vi "HOST_UIC1203R.vi"() -> ()   [LabVIEW 2018]
uses:
  <instrlib>/niFgen/niFgen.llb/niFgen Output Mode.ctl
  <instrlib>/niDMM/nidmm.llb/niDMM Function.ctl
  <instrlib>/niDCPower/nidcpower.llb/niDCPower Measurement Type.ctl
  <instrlib>/niDMM/nidmm.llb/niDMM Configure Measurement Absolute.vi
panel:
  out "Power, мВт":dbl
  in  "Генератор":bool
  in  "Standard Waveform":u16(slide)=1 scale=0.0..6.0
  in  "Frequency (Hz)":dbl(knob)=50.0 min=1.0 max=100000000.0 scale=0.0..100000000.0 scale format="%_1p"
  in  "Amplitude (Vp-p)":dbl(knob)=2.4999999999999996 min=0.0 max=12.0 scale=0.0..12.0 scale format="%.1f"
  in  "DC Offset (V)":dbl(knob)=0.2 min=-6.0 max=6.0 scale=-6.0..6.0 scale format="%_1p"
  in  "FGEN Resource Name":refnum<k15>="Dev1"
  out "SEU, мВ":dbl
  in  "Instrument Descriptor":refnum<k15>="PXI1Slot5"
  in  "Питание":bool
  out "Номер образца":string="0"
  in  "SEL":path=path "C:/LabView_PRJ/23011_UIC1203R/LabView_PRJ/SEL"
  in  "DVDD_VDDA":refnum<k15>="PXI1Slot4" caption="instrument handle"
  in  "VDPIX_VCC":refnum<k15>="PXI1Slot3" caption="instrument handle"
  in  "VDA_VDD":refnum<k15>="PXI1Slot2" caption="instrument handle"
  out "VDDA Chart":dbl(graph)=0.0007214157137472484 caption="Waveform Chart 5"
  out "VDDA_cur, A":dbl caption="measurement" format="%_6g"
  in  "VDDA_curlim, A":dbl=0.1 caption="current limit" format="%_6p"
  in  "VDDA, V":dbl=1.8 caption="voltage level" format="%_6p"
  out "DVDD Chart":dbl(graph)=0.10338513624280214 caption="Waveform Chart 5"
  out "DVDD_cur, A":dbl caption="measurement" format="%_6g"
  in  "DVDD_curlim, A":dbl=0.1 caption="current limit" format="%_6p"
  in  "DVDD, V":dbl=3.3 caption="voltage level" format="%_6p"
  out "VCC Chart":dbl(graph)=-0.0011085533359822216
  out "VCC_cur, A":dbl caption="measurement" format="%_6g"
  in  "VCC, V":dbl=3.3 caption="voltage level" format="%_6p"
  in  "VCC_curlim, A":dbl=0.1 caption="current limit" format="%_6p"
  out "VDA Chart":dbl(graph)=-0.15026988538913832 caption="Waveform Chart 5"
  out "VDPIX Chart":dbl(graph)=0.2888581876247902
  out "VDD Chart":dbl(graph)=-0.0007912650485297681
  out "VDPIX_cur, A":dbl caption="measurement" format="%_6g"
  in  "VDPIX_curlim, A":dbl=0.1 caption="current limit" format="%_6p"
  in  "VDPIX, V":dbl=1.8 caption="voltage level" format="%_6p"
  in  "VDD, V":dbl=1.8 caption="voltage level" format="%_6p"
  out "VDD_cur, A":dbl caption="measurement" format="%_6g"
  out "VDA_cur, A":dbl caption="measurement" format="%_6g"
  in  "VDD_curlim, A":dbl=0.1 caption="current limit" format="%_6p"
  in  "VDA_curlim, A":dbl=0.1 caption="current limit" format="%_6p"
  in  "VDA, V":dbl=1.8 caption="voltage level" format="%_6p"
  in  "Стоп":bool
  in  "Период, мс":u32=100
  out "DVDD":bool
  out "DVDD":i32
  in  "DVDD_selcur":dbl=0.095 caption="current limit" format="%_6p"
  out "VCC":bool
  out "VCC":i32
  in  "VCC_selcur":dbl=0.095 caption="current limit" format="%_6p"
  out "VDPIX":bool
  out "VDPIX":i32
  out "VDD":bool
  out "VDD":i32
  out "VDA":bool
  out "VDA":i32
  in  "VDPIX_selcur":dbl=0.095 caption="current limit" format="%_6p"
  in  "VDD_selcur":dbl=0.095 caption="current limit" format="%_6p"
  in  "VDA_selcur":dbl=0.095 caption="current limit" format="%_6p"
  out "SEL":bool
  in  "SIM_SEL":bool
  out "VDDA":bool
  out "VDDA":i32
  in  "VDDA_selcur":dbl=0.095 caption="current limit" format="%_6p"
  # "2"
  # "1"
  # "3"
  # "Гц"
  # "Амплитуда"
  # "Смещение"
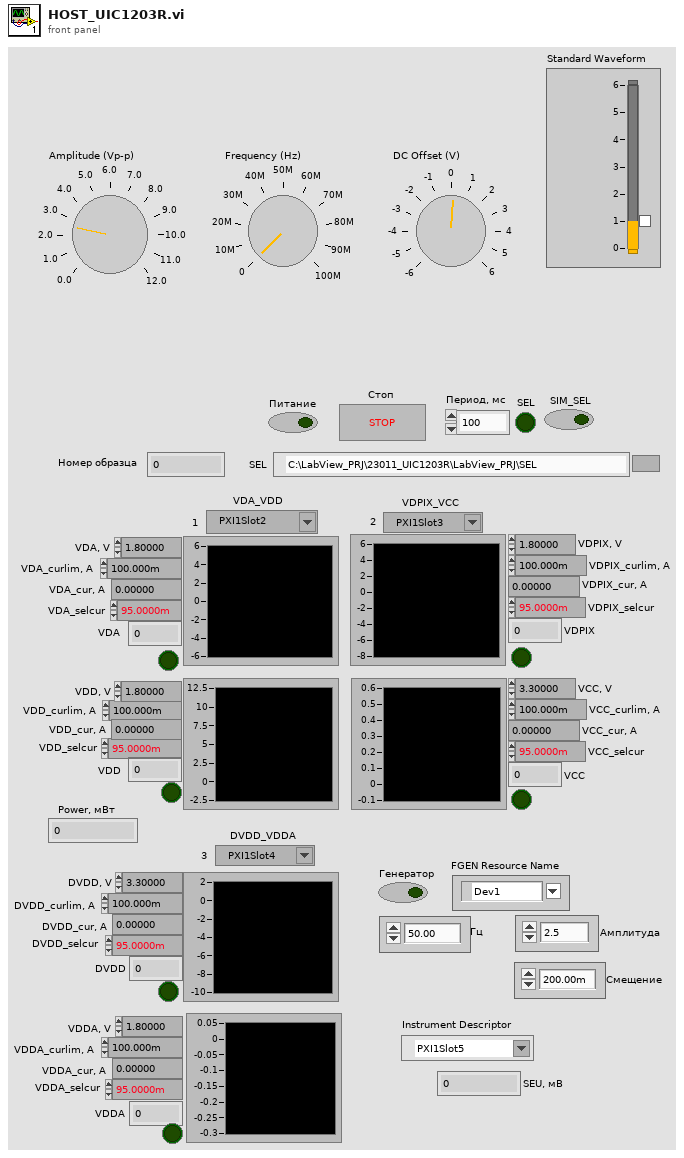
[diagram p1: front panel]
types:
  T1 = typedef "niFgen Output Mode.ctl" = u32
  T2 = enum16{"open", "replace", "create", "open or create", "replace or create", "replace or create with confirmation"}
  T3 = typedef "niDCPower Measurement Type.ctl" = i32
  T4 = typedef "niDMM Function.ctl" = enum16{"DC Volts", "AC Volts", "DC Current", "AC Current", "2-wire Resistance", "4-wire Resistance", "Diode", "Frequency", "Period", "AC Volts DC Coupled", "Capacitance", "Inductance", "Temperature"}
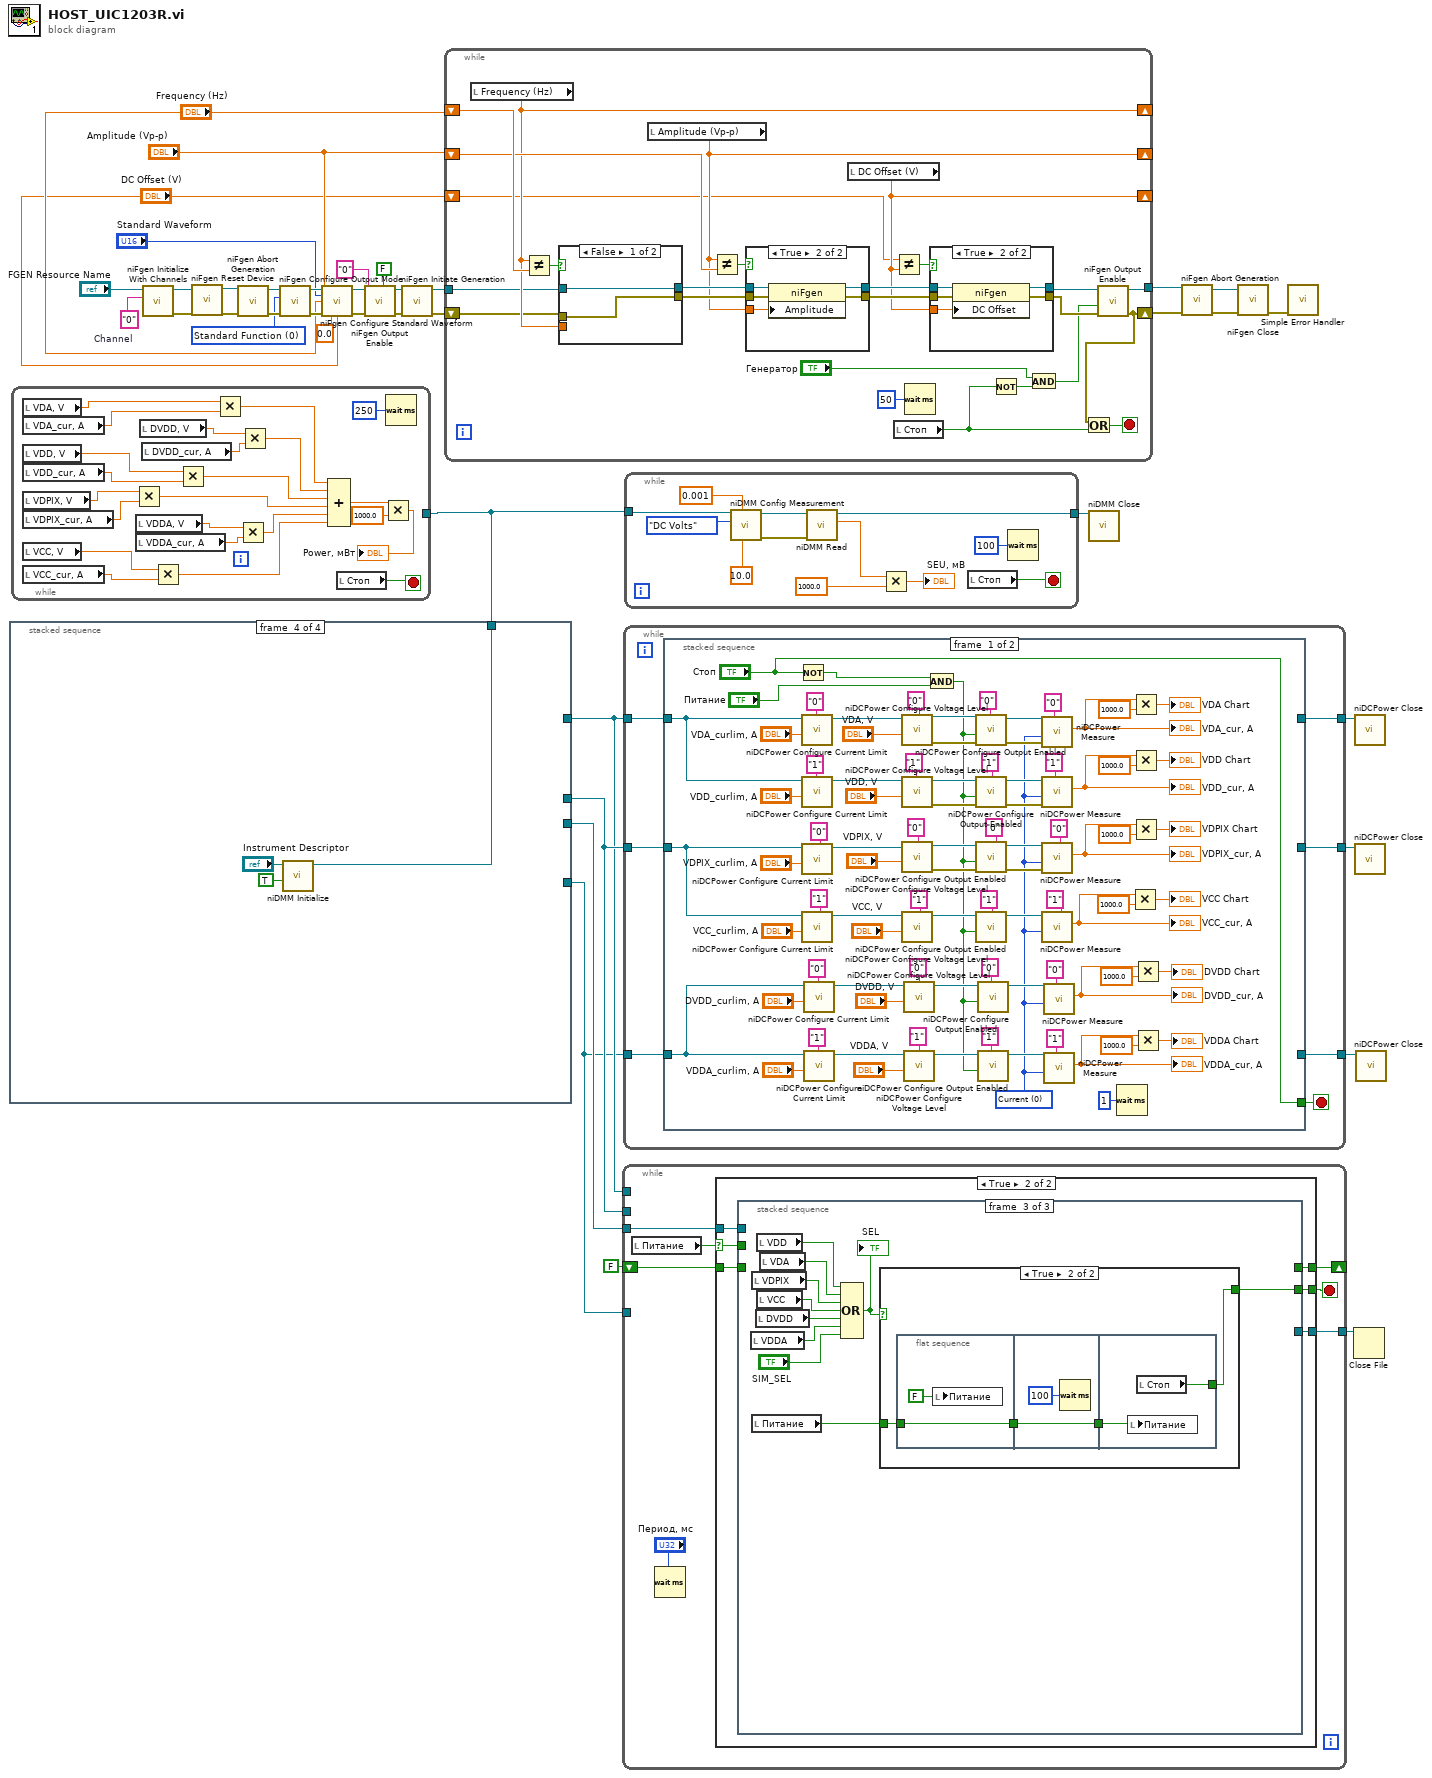
[diagram p0: block diagram]
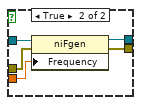
[diagram p4: hidden frame]
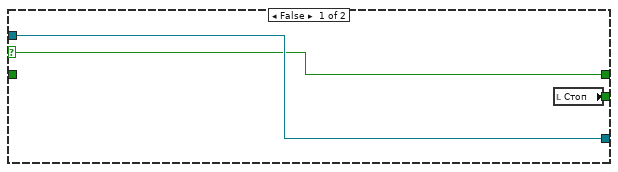
[diagram p5: hidden frame]
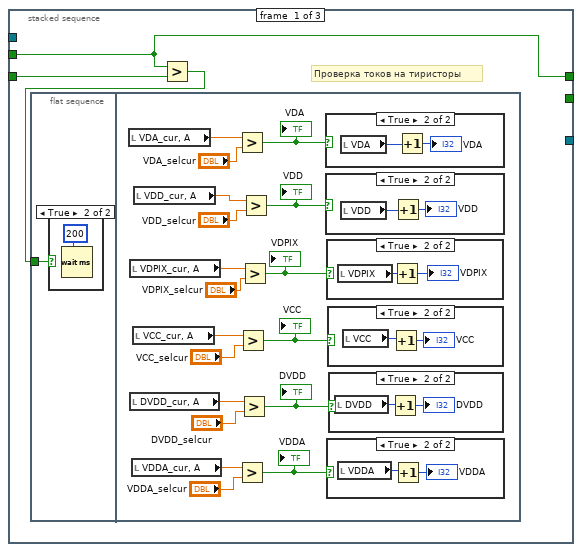
[diagram p6: hidden frame]
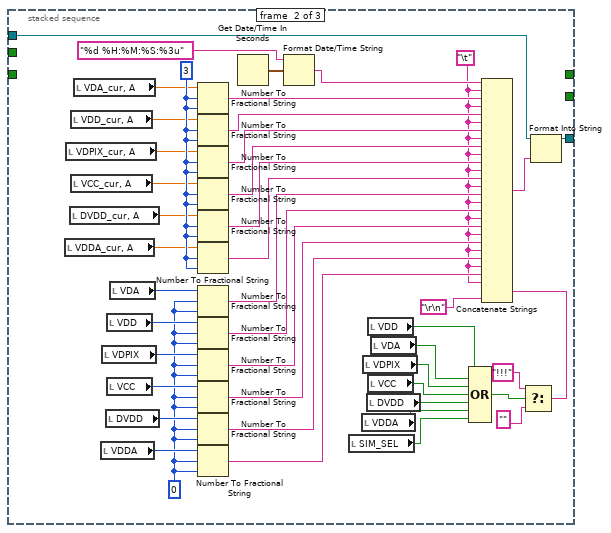
[diagram p14: hidden frame]
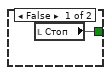
[diagram p15: hidden frame]
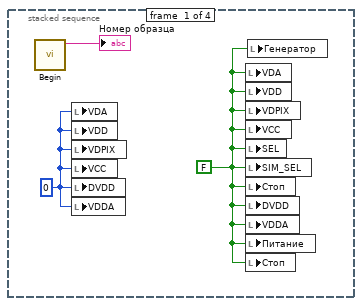
[diagram p17: hidden frame]
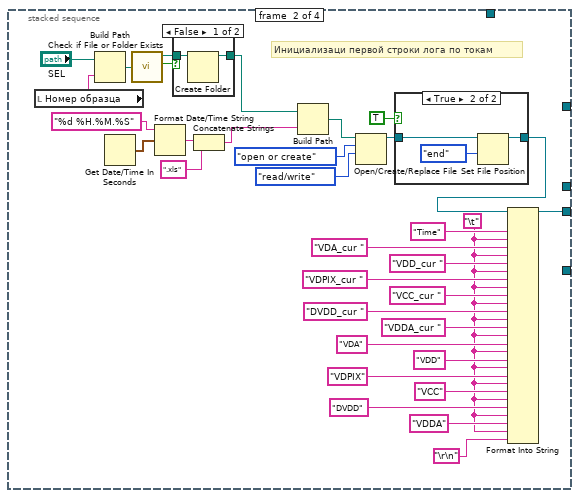
[diagram p18: hidden frame]
diagram:
  w20 = T1 0 items=["Standard Function", "Frequency List", "Arbitrary Waveform", "Arbitrary Sequence", "Script"] ("output mode")
  w9 = "0"  # Channel
  n1 = stacked-sequence {
    tunnel: [_ _ w94 _] -> w37
    tunnel: [_ _ w93 _] -> w36
    tunnel: [_ w60 _ _] -> w39
    tunnel: [_ _ w87 _] -> w32
    tunnel: [_ _ _ w105] -> w1
    frame #0 {
      w42 = 0
      w41 = FALSE
      n2 = call "Begin.vi"() -> ("Номер образца 2"=→"Номер образца":string)  [unwired: 11 in]
      n3 = local write "VDA"(w42) -> ()
      n4 = local write "VDD"(w42) -> ()
      n5 = local write "VDPIX"(w42) -> ()
      n6 = local write "VCC"(w42) -> ()
      n7 = local write "DVDD"(w42) -> ()
      n8 = local write "VDDA"(w42) -> ()
      n9 = local write "VDA"(w41) -> ()
      n10 = local write "VDD"(w41) -> ()
      n11 = local write "VDPIX"(w41) -> ()
      n12 = local write "VCC"(w41) -> ()
      n13 = local write "SEL"(w41) -> ()
      n14 = local write "SIM_SEL"(w41) -> ()
      n15 = local write "Стоп"(w41) -> ()
      n16 = local write "DVDD"(w41) -> ()
      n17 = local write "VDDA"(w41) -> ()
      n18 = local write "Питание"(w41) -> ()
      n19 = local write "Стоп"(w41) -> ()
      n20 = local write "Генератор"(w41) -> ()
    }
    frame #1 {
      w45 = "\t"
      # "Инициализаци первой строки лога по токам"
      n21 = local read "Номер образца"() -> (w72:string)
      n22 = Build Path(base path="SEL", name or relative path=w72) -> (appended path=w74:path)
      n23 = Get Date/Time In Seconds() -> (seconds since 1Jan1904=w67:timestamp)
      n24 = call <vilib>:"Check if File or Folder Exists.vi"("path"=w74) -> ("file or folder exists?"=w75:bool, "dup path"=w76:path)  [unwired: 8 in, 1 out]
      n25 = Format Date/Time String(time format string (%c)="%d %H.%M.%S", seconds (now)=w67) -> (date/time string=w64:string)  [unwired: 1 in]
      n26 = case shown="False" w75 {
        tunnel: w76 -> [w82 w83]
        tunnel: [w81 w83] -> w59
        frame False {
          n27 = Create Folder(path (use dialog)=w82) -> (created path=w81:path)  [unwired: 2 in, 2 out]
        }
        frame True {
        }
      }
      n28 = Concatenate Strings(w64, ".xls" ("string")) -> (w62:string)
      n29 = Build Path(base path=w59, name or relative path=w62) -> (appended path=w65:path)
      n30 = Open/Create/Replace File(file path (use dialog)=w65, operation (0:open)=T2."open or create", access (0:read/write)=enum16{"read/write", "read-only", "write-only"}."read/write") -> (refnum out=w68:refnum<file>)  [unwired: 3 in, 2 out]
      n31 = case shown="True" TRUE {
        tunnel: w68 -> [w77 w80]
        tunnel: [w77 w78] -> w61
        frame False {
        }
        frame True {
          n32 = Set File Position(refnum=w80, from (0:start)=enum16{"start", "end", "current"}."end") -> (refnum out=w78:refnum<file>)  [unwired: 2 in, 1 out]
        }
      }
      n33 = Format Into String(initial string=w61, "Time" ("input 1"), w45, "VDA_cur " ("input 1"), w45, "VDD_cur " ("input 1"), w45, "VDPIX_cur " ("input 1"), w45, "VCC_cur " ("input 1"), w45, "DVDD_cur " ("input 1"), w45, "VDDA_cur " ("input 1"), w45, "VDA" ("input 1"), w45, "VDD" ("input 1"), w45, "VDPIX" ("input 1"), w45, "VCC" ("input 1"), w45, "DVDD" ("input 1"), w45, "VDDA" ("input 1"), w45, "\r\n") -> (resulting string=w60:refnum<file>)  [unwired: 2 in, 1 out]
    }
    frame #2 {
      n34 = call <instrlib>:"niDCPower Initialize.vi"("reset device"=TRUE, "resource name"="DVDD_VDDA") -> ("error out"=w90:errorcluster, "instrument handle out"=w89:refnum<k15>)  [unwired: 2 in, 6 out]
      n35 = call <instrlib>:"niDCPower Initialize.vi"("reset device"=TRUE, "resource name"="VDA_VDD") -> ("error out"=w101:errorcluster, "instrument handle out"=w103:refnum<k15>)  [unwired: 2 in, 6 out]
      n36 = call <instrlib>:"niDCPower Initialize.vi"("reset device"=TRUE, "resource name"="VDPIX_VCC") -> ("error out"=w102:errorcluster, "instrument handle out"=w104:refnum<k15>)  [unwired: 2 in, 6 out]
      n37 = call <instrlib>:"niDCPower Configure Voltage Level.vi"("error in (no error)"=w101, "voltage level"=0.0, "channel name"="0,1", "instrument handle"=w103) -> ("instrument handle out"=w93:refnum<k15>)  [unwired: 6 in, 1 out]
      n38 = call <instrlib>:"niDCPower Configure Voltage Level.vi"("error in (no error)"=w102, "voltage level"=0.0, "channel name"="0,1", "instrument handle"=w104) -> ("instrument handle out"=w94:refnum<k15>)  [unwired: 6 in, 1 out]
      n39 = call <instrlib>:"niDCPower Configure Voltage Level.vi"("error in (no error)"=w90, "voltage level"=0.0, "channel name"="0,1", "instrument handle"=w89) -> ("instrument handle out"=w87:refnum<k15>)  [unwired: 6 in, 1 out]
    }
    frame #3 {
      n40 = call <instrlib>:"niDMM Initialize.vi"("Reset"=TRUE, "Instrument Descriptor"="Instrument Descriptor") -> ("instrument handle out"=w105:refnum<k15>)  [unwired: 8 in, 1 out]
    }
  }
  n41 = while {
    tunnel: w1 -> [_]
    stop <- w130 stop-if-true
    n42 = local read "VDA, V"() -> (w126:dbl)
    n43 = local read "VDA_cur, A"() -> (w125:dbl)
    n44 = local read "VDD, V"() -> (w122:dbl)
    n45 = local read "VDD_cur, A"() -> (w121:dbl)
    n46 = local read "VDPIX, V"() -> (w127:dbl)
    n47 = local read "VDPIX_cur, A"() -> (w128:dbl)
    n48 = local read "VCC, V"() -> (w120:dbl)
    n49 = local read "VCC_cur, A"() -> (w119:dbl)
    n50 = Multiply(x=w127, y=w128) -> (x*y=w113:dbl)
    n51 = local read "VDDA, V"() -> (w118:dbl)
    n52 = local read "VDDA_cur, A"() -> (w117:dbl)
    n53 = local read "DVDD, V"() -> (w124:dbl)
    n54 = local read "DVDD_cur, A"() -> (w123:dbl)
    n55 = Multiply(x=w120, y=w119) -> (x*y=w111:dbl)
    n56 = Multiply(x=w122, y=w121) -> (x*y=w114:dbl)
    n57 = Multiply(x=w126, y=w125) -> (x*y=w116:dbl)
    n58 = Multiply(x=w118, y=w117) -> (x*y=w112:dbl)
    n59 = Multiply(x=w124, y=w123) -> (x*y=w115:dbl)
    n60 = Compound Arithmetic op=ADD(w116, w115, w114, w113, w112, w111) -> (w110:dbl)
    n61 = local read "Стоп"() -> (w130:bool)
    n62 = Multiply(x=w110, y=1000.0) -> (x*y=→"Power, мВт":dbl)
    n63 = Wait (ms)(milliseconds to wait=u32 250) -> ()  [unwired: 1 out]
  }
  n64 = call <instrlib>:"niFgen Initialize With Channels.vi"("Channel Name"=w9, "Resource Name"="FGEN Resource Name") -> ("error out"=w2:errorcluster, "Instrument Handle Out"=w5:refnum<k15>)  [unwired: 8 in]
  n65 = call <instrlib>:"niFgen Reset Device.vi"("error in (no error)"=w2, "Instrument Handle"=w5) -> ("error out"=w3:errorcluster, "Instrument Handle Out"=w4:refnum<k15>)  [unwired: 8 in]
  n66 = call <instrlib>:"niFgen Abort Generation.vi"("error in (no error)"=w3, "Instrument Handle"=w4) -> ("error out"=w23:errorcluster, "Instrument Handle Out"=w22:refnum<k15>)  [unwired: 8 in]
  n67 = call <instrlib>:"niFgen Configure Output Mode.vi"("error in (no error)"=w23, "Output Mode (default: 0=Standard Function)"=w20, "Instrument Handle"=w22) -> ("error out"=w27:errorcluster, "Instrument Handle Out"=w25:refnum<k15>)  [unwired: 6 in]
  n68 = call <instrlib>:"niFgen Configure Standard Waveform.vi"("Instrument Handle"=w25, "Waveform"="Standard Waveform", "Frequency"="Frequency (Hz)", "Amplitude"="Amplitude (Vp-p)", "error in (no error)"=w27, "Start Phase"=0.0, "DC Offset"="DC Offset (V)") -> ("Instrument Handle Out"=w18:refnum<k15>, "error out"=w19:errorcluster)  [unwired: 7 in]
  n69 = call <instrlib>:"niFgen Output Enable.vi"("error in (no error)"=w19, "Output Enable (default: True)"=FALSE ("output enable"), "Channel Name"="0", "Instrument Handle"=w18) -> ("error out"=w26:errorcluster, "Instrument Handle Out"=w24:refnum<k15>)  [unwired: 6 in]
  n70 = call <instrlib>:"niFgen Initiate Generation.vi"("error in (no error)"=w26, "Instrument Handle"=w24) -> ("error out"=w13:errorcluster, "Instrument Handle Out"=w17:refnum<k15>)  [unwired: 8 in]
  n71 = while {
    tunnel: w17 -> [w131]
    tunnel: [w140] -> w16
    shift-right: [w144] -> _
    shift-left: "Frequency (Hz)" -> [w151]
    shift-right: [w143] -> _
    shift-left: "Amplitude (Vp-p)" -> [w150]
    shift-right: [w142] -> _
    shift-left: "DC Offset (V)" -> [w141]
    shift-right: [w136] -> w12
    shift-left: w13 -> [w132]
    stop <- w145 stop-if-true
    n72 = local read "Frequency (Hz)"() -> (w144:dbl)
    n73 = Not Equal?(x=w144, y=w151) -> (x != y?=w149:bool)
    n74 = case shown="False" w149 {
      tunnel: [w171 w176] -> w152
      tunnel: [w170 w175] -> w153
      tunnel: w131 -> [w171 w174]
      tunnel: w144 -> [_ w173]
      tunnel: w132 -> [w170 w172]
      frame False {
      }
      frame True {
        n75 = property class="niFgen"(reference=w174, error in=w172, "Frequency"=w173) -> (reference out=w176:refnum<k15>, error out=w175:errorcluster)
      }
    }
    n76 = local read "Amplitude (Vp-p)"() -> (w143:dbl)
    n77 = Not Equal?(x=w143, y=w150) -> (x != y?=w148:bool)
    n78 = case shown="True" w148 {
      tunnel: w152 -> [w164 w169]
      tunnel: w153 -> [w163 w168]
      tunnel: [w163 w167] -> w154
      tunnel: [w164 w166] -> w155
      tunnel: w143 -> [_ w165]
      frame False {
      }
      frame True {
        n79 = property class="niFgen"(reference=w169, error in=w168, "Amplitude"=w165) -> (reference out=w166:refnum<k15>, error out=w167:errorcluster)
      }
    }
    n80 = local read "DC Offset (V)"() -> (w142:dbl)
    n81 = Not Equal?(x=w141, y=w142) -> (x != y?=w147:bool)
    n82 = local read "Стоп"() -> (w134:bool)
    n83 = Wait (ms)(milliseconds to wait=u32 50) -> ()  [unwired: 1 out]
    n84 = case shown="True" w147 {
      tunnel: w154 -> [w156 w162]
      tunnel: w155 -> [w157 w161]
      tunnel: [w157 w160] -> w139
      tunnel: [w156 w159] -> w138
      tunnel: w142 -> [_ w158]
      frame False {
      }
      frame True {
        n85 = property class="niFgen"(reference=w161, error in=w162, "DC Offset"=w158) -> (reference out=w160:refnum<k15>, error out=w159:errorcluster)
      }
    }
    n86 = Not(x=w134) -> (.not. x?=w137:bool)
    n87 = And(x="Генератор", y=w137) -> (x .and. y?=w133:bool)
    n88 = call <instrlib>:"niFgen Output Enable.vi"("error in (no error)"=w138, "Output Enable (default: True)"=w133, "Instrument Handle"=w139) -> ("error out"=w136:errorcluster, "Instrument Handle Out"=w140:refnum<k15>)  [unwired: 7 in]
    n89 = Or(x=w136, y=w134) -> (x .or. y?=w145:bool)
  }
  n90 = while {
    shift-right: [w177] -> _
    shift-left: FALSE -> [w183]
    tunnel: w39 -> [w182]
    tunnel: [w180] -> w38
    tunnel: w32 -> [_]
    tunnel: w37 -> [_]
    tunnel: w36 -> [_]
    stop <- w181 stop-if-true
    n91 = local read "Питание"() -> (w178:bool)
    n92 = Wait (ms)(milliseconds to wait="Период, мс") -> ()  [unwired: 1 out]
    n93 = case shown="True" w178 {
      selector: w178 -> [w184 w188]
      tunnel: w183 -> [_ w192]
      tunnel: w182 -> [w185 w191]
      tunnel: [w186 w190] -> w181
      tunnel: [w185 w189] -> w180
      tunnel: [w184 w187] -> w177
      frame False {
        n94 = local read "Стоп"() -> (w186:bool)
      }
      frame True {
        n95 = stacked-sequence {
          tunnel: w192 -> [w195 _ _]
          tunnel: w191 -> [_ w262 _]
          tunnel: [_ _ w274] -> w190
          tunnel: [_ w260 _] -> w189
          tunnel: w188 -> [w194 _ _]
          tunnel: [w194 _ _] -> w187
          frame #0 {
            # "Проверка токов на тиристоры"
            n96 = flat-sequence {
              tunnel: w193 -> [w196]
              frame #0 {
                n97 = case shown="True" w196 {
                  frame False {
                  }
                  frame True {
                    n98 = Wait (ms)(milliseconds to wait=u32 200) -> ()  [unwired: 1 out]
                  }
                }
              }
              frame #1 {
                n99 = local read "VDA_cur, A"() -> (w209:dbl)
                n100 = local read "VDPIX_cur, A"() -> (w207:dbl)
                n101 = local read "DVDD_cur, A"() -> (w201:dbl)
                n102 = local read "VDDA_cur, A"() -> (w198:dbl)
                n103 = local read "VCC_cur, A"() -> (w206:dbl)
                n104 = local read "VDD_cur, A"() -> (w208:dbl)
                n105 = Greater?(x=w209, y="VDA_selcur") -> (0:w214:bool)
                "VDA" <- w214
                n106 = Greater?(x=w198, y="VDDA_selcur") -> (0:w200:bool)
                "VDDA" <- w200
                n107 = Greater?(x=w206, y="VCC_selcur") -> (0:w205:bool)
                "VCC" <- w205
                n108 = Greater?(x=w201, y="DVDD_selcur") -> (0:w202:bool)
                "DVDD" <- w202
                n109 = Greater?(x=w207, y="VDPIX_selcur") -> (0:w210:bool)
                "VDPIX" <- w210
                n110 = Greater?(x=w208, y="VDD_selcur") -> (0:w212:bool)
                "VDD" <- w212
                n111 = case shown="True" w214 {
                  frame False {
                  }
                  frame True {
                    n112 = local read "VDA"() -> (w227:i32)
                    n113 = Increment(x=w227) -> (x+1=→"VDA":i32)
                  }
                }
                n114 = case shown="True" w212 {
                  frame False {
                  }
                  frame True {
                    n115 = local read "VDD"() -> (w224:i32)
                    n116 = Increment(x=w224) -> (x+1=→"VDD":i32)
                  }
                }
                n117 = case shown="True" w210 {
                  frame False {
                  }
                  frame True {
                    n118 = local read "VDPIX"() -> (w223:i32)
                    n119 = Increment(x=w223) -> (x+1=→"VDPIX":i32)
                  }
                }
                n120 = case shown="True" w200 {
                  frame False {
                  }
                  frame True {
                    n121 = local read "VDDA"() -> (w217:i32)
                    n122 = Increment(x=w217) -> (x+1=→"VDDA":i32)
                  }
                }
                n123 = case shown="True" w205 {
                  frame False {
                  }
                  frame True {
                    n124 = local read "VCC"() -> (w221:i32)
                    n125 = Increment(x=w221) -> (x+1=→"VCC":i32)
                  }
                }
                n126 = case shown="True" w202 {
                  frame False {
                  }
                  frame True {
                    n127 = local read "DVDD"() -> (w219:i32)
                    n128 = Increment(x=w219) -> (x+1=→"DVDD":i32)
                  }
                }
              }
            }
            n129 = Greater?(x=w194, y=w195) -> (0:w193:bool)
          }
          frame #1 {
            w230 = i16 0 ("width (-)")
            w259 = i16 3 ("width (-)")
            w231 = "\t"
            n130 = local read "VDDA_cur, A"() -> (w250:dbl)
            n131 = local read "VDPIX_cur, A"() -> (w253:dbl)
            n132 = local read "DVDD_cur, A"() -> (w251:dbl)
            n133 = local read "VDD_cur, A"() -> (w254:dbl)
            n134 = local read "VCC_cur, A"() -> (w252:dbl)
            n135 = local read "VDA_cur, A"() -> (w255:dbl)
            n136 = local read "VDDA"() -> (w240:i32)
            n137 = local read "VDPIX"() -> (w247:i32)
            n138 = local read "DVDD"() -> (w245:i32)
            n139 = local read "VDD"() -> (w248:i32)
            n140 = local read "VCC"() -> (w246:i32)
            n141 = local read "VDA"() -> (w249:i32)
            n142 = Number To Fractional String(number=w255, width (-)=w259, precision (6)=w259) -> (F-format string=w266:string)  [unwired: 1 in]
            n143 = Number To Fractional String(number=w254, width (-)=w259, precision (6)=w259) -> (F-format string=w265:string)  [unwired: 1 in]
            n144 = Number To Fractional String(number=w253, width (-)=w259, precision (6)=w259) -> (F-format string=w264:string)  [unwired: 1 in]
            n145 = Number To Fractional String(number=w252, width (-)=w259, precision (6)=w259) -> (F-format string=w261:string)  [unwired: 1 in]
            n146 = Number To Fractional String(number=w251, width (-)=w259, precision (6)=w259) -> (F-format string=w257:string)  [unwired: 1 in]
            n147 = Number To Fractional String(number=w250, width (-)=w259, precision (6)=w259) -> (F-format string=w256:string)  [unwired: 1 in]
            n148 = Number To Fractional String(number=w249, width (-)=w230, precision (6)=w230) -> (F-format string=w237:string)  [unwired: 1 in]
            n149 = Number To Fractional String(number=w248, width (-)=w230, precision (6)=w230) -> (F-format string=w236:string)  [unwired: 1 in]
            n150 = Number To Fractional String(number=w247, width (-)=w230, precision (6)=w230) -> (F-format string=w235:string)  [unwired: 1 in]
            n151 = Number To Fractional String(number=w246, width (-)=w230, precision (6)=w230) -> (F-format string=w234:string)  [unwired: 1 in]
            n152 = Number To Fractional String(number=w245, width (-)=w230, precision (6)=w230) -> (F-format string=w233:string)  [unwired: 1 in]
            n153 = Number To Fractional String(number=w240, width (-)=w230, precision (6)=w230) -> (F-format string=w232:string)  [unwired: 1 in]
            n154 = Get Date/Time In Seconds() -> (seconds since 1Jan1904=w272:timestamp)
            n155 = Format Date/Time String(time format string (%c)="%d %H:%M:%S:%3u", seconds (now)=w272) -> (date/time string=w267:string)  [unwired: 1 in]
            n156 = local read "SIM_SEL"() -> (w238:bool)
            n157 = local read "VDDA"() -> (w239:bool)
            n158 = local read "VDPIX"() -> (w242:bool)
            n159 = local read "DVDD"() -> (w258:bool)
            n160 = local read "VDD"() -> (w244:bool)
            n161 = local read "VCC"() -> (w241:bool)
            n162 = local read "VDA"() -> (w243:bool)
            n163 = Compound Arithmetic op=OR(w244, w243, w242, w241, w258, w239, w238) -> (w263:bool)
            n164 = Select(t="!!!", s=w263, f="") -> (s? t:f=w229:string)
            n165 = Concatenate Strings(w267, w231, w266, w231, w265, w231, w264, w231, w261, w231, w257, w231, w256, w231, w237, w231, w236, w231, w235, w231, w234, w231, w233, w231, w232, w231, w229, "\r\n") -> (w271:string)
            n166 = Format Into String(initial string=w262, w271) -> (resulting string=w260:refnum<file>)  [unwired: 2 in, 1 out]
          }
          frame #2 {
            n167 = local read "VDDA"() -> (w276:bool)
            n168 = local read "VDPIX"() -> (w278:bool)
            n169 = local read "Питание"() -> (w273:bool)
            n170 = local read "DVDD"() -> (w282:bool)
            n171 = local read "VDD"() -> (w280:bool)
            n172 = local read "VCC"() -> (w277:bool)
            n173 = local read "VDA"() -> (w279:bool)
            n174 = Compound Arithmetic op=OR(w280, w279, w278, w277, w282, w276, "SIM_SEL") -> (w281:bool)
            "SEL" <- w281
            n175 = case shown="True" w281 {
              tunnel: [w283 w284] -> w274
              tunnel: w273 -> [_ w285]
              frame False {
                n176 = local read "Стоп"() -> (w283:bool)
              }
              frame True {
                n177 = flat-sequence {
                  tunnel: [w288] -> w286
                  tunnel: w285 -> [w288]
                  tunnel: [w290] -> w287
                  tunnel: w286 -> [w290]
                  tunnel: w287 -> [w293]
                  tunnel: [w292] -> w284
                  frame #0 {
                    n178 = local write "Питание"(FALSE ("Питание")) -> ()
                  }
                  frame #1 {
                    n179 = Wait (ms)(milliseconds to wait=u32 100) -> ()  [unwired: 1 out]
                  }
                  frame #2 {
                    n180 = local write "Питание"(w293) -> ()
                    n181 = local read "Стоп"() -> (w292:bool)
                  }
                }
              }
            }
          }
        }
      }
    }
  }
  n182 = while {
    tunnel: w36 -> [w300]
    tunnel: w32 -> [w298]
    tunnel: w37 -> [w299]
    tunnel: [w297] -> w35
    tunnel: [w296] -> w34
    tunnel: [w295] -> w33
    stop <- w294 stop-if-true
    n183 = stacked-sequence {
      tunnel: w298 -> [w307 w388]
      tunnel: w299 -> [w306 w389]
      tunnel: w300 -> [w305 w390]
      tunnel: [_ w390] -> w297
      tunnel: [_ w389] -> w296
      tunnel: [_ w388] -> w295
      tunnel: ["Стоп" _] -> w294
      frame #0 {
        w308 = T3 0 items=["Current", "Voltage"] ("measurement type")
        n184 = Not(x="Стоп") -> (.not. x?=w302:bool)
        n185 = call <instrlib>:"niDCPower Configure Current Limit.vi"("current limit"="VDA_curlim, A", "channel name"="0", "instrument handle"=w305) -> ("instrument handle out"=w376:refnum<k15>)  [unwired: 7 in, 1 out]
        n186 = call <instrlib>:"niDCPower Configure Current Limit.vi"("current limit"="VDD_curlim, A", "channel name"="1", "instrument handle"=w305) -> ("instrument handle out"=w377:refnum<k15>)  [unwired: 7 in, 1 out]
        n187 = call <instrlib>:"niDCPower Configure Current Limit.vi"("current limit"="VDPIX_curlim, A", "channel name"="0", "instrument handle"=w306) -> ("instrument handle out"=w359:refnum<k15>)  [unwired: 7 in, 1 out]
        n188 = call <instrlib>:"niDCPower Configure Current Limit.vi"("current limit"="VCC_curlim, A", "channel name"="1", "instrument handle"=w306) -> ("instrument handle out"=w339:refnum<k15>)  [unwired: 7 in, 1 out]
        n189 = call <instrlib>:"niDCPower Configure Current Limit.vi"("current limit"="DVDD_curlim, A", "channel name"="0", "instrument handle"=w307) -> ("instrument handle out"=w330:refnum<k15>)  [unwired: 7 in, 1 out]
        n190 = call <instrlib>:"niDCPower Configure Current Limit.vi"("current limit"="VDDA_curlim, A", "channel name"="1", "instrument handle"=w307) -> ("instrument handle out"=w311:refnum<k15>)  [unwired: 7 in, 1 out]
        n191 = call <instrlib>:"niDCPower Configure Voltage Level.vi"("voltage level"="VDA, V", "channel name"="0", "instrument handle"=w376) -> ("error out"=w369:errorcluster, "instrument handle out"=w372:refnum<k15>)  [unwired: 7 in]
        n192 = call <instrlib>:"niDCPower Configure Voltage Level.vi"("voltage level"="VDD, V", "channel name"="1", "instrument handle"=w377) -> ("error out"=w370:errorcluster, "instrument handle out"=w371:refnum<k15>)  [unwired: 7 in]
        n193 = call <instrlib>:"niDCPower Configure Voltage Level.vi"("voltage level"="VDPIX, V", "channel name"="0", "instrument handle"=w359) -> ("error out"=w363:errorcluster, "instrument handle out"=w364:refnum<k15>)  [unwired: 7 in]
        n194 = call <instrlib>:"niDCPower Configure Voltage Level.vi"("voltage level"="VCC, V", "channel name"="1", "instrument handle"=w339) -> ("instrument handle out"=w337:refnum<k15>)  [unwired: 7 in, 1 out]
        n195 = call <instrlib>:"niDCPower Configure Voltage Level.vi"("voltage level"="DVDD, V", "channel name"="0", "instrument handle"=w330) -> ("instrument handle out"=w329:refnum<k15>)  [unwired: 7 in, 1 out]
        n196 = call <instrlib>:"niDCPower Configure Voltage Level.vi"("voltage level"="VDDA, V", "channel name"="1", "instrument handle"=w311) -> ("instrument handle out"=w312:refnum<k15>)  [unwired: 7 in, 1 out]
        n197 = And(x=w302, y="Питание") -> (x .and. y?=w303:bool)
        n198 = call <instrlib>:"niDCPower Configure Output Enabled.vi"("error in (no error)"=w369, "output enabled"=w303, "channel name"="0", "instrument handle"=w372) -> ("error out"=w381:errorcluster, "instrument handle out"=w380:refnum<k15>)  [unwired: 6 in]
        n199 = call <instrlib>:"niDCPower Configure Output Enabled.vi"("error in (no error)"=w370, "output enabled"=w303, "channel name"="1", "instrument handle"=w371) -> ("error out"=w382:errorcluster, "instrument handle out"=w383:refnum<k15>)  [unwired: 6 in]
        n200 = call <instrlib>:"niDCPower Configure Output Enabled.vi"("error in (no error)"=w363, "output enabled"=w303, "channel name"="0", "instrument handle"=w364) -> ("error out"=w355:errorcluster, "instrument handle out"=w356:refnum<k15>)  [unwired: 6 in]
        n201 = call <instrlib>:"niDCPower Configure Output Enabled.vi"("output enabled"=w303, "channel name"="1", "instrument handle"=w337) -> ("instrument handle out"=w335:refnum<k15>)  [unwired: 7 in, 1 out]
        n202 = call <instrlib>:"niDCPower Configure Output Enabled.vi"("output enabled"=w303, "channel name"="0", "instrument handle"=w329) -> ("instrument handle out"=w328:refnum<k15>)  [unwired: 7 in, 1 out]
        n203 = call <instrlib>:"niDCPower Configure Output Enabled.vi"("output enabled"=w303, "channel name"="1", "instrument handle"=w312) -> ("instrument handle out"=w313:refnum<k15>)  [unwired: 7 in, 1 out]
        n204 = call <instrlib>:"niDCPower Measure.vi"("error in (no error)"=w381, "measurement type"=w308, "channel name"="0", "instrument handle"=w380) -> ("measurement"=w348:dbl)  [unwired: 5 in, 2 out]
        "VDA_cur, A" <- w348
        n205 = call <instrlib>:"niDCPower Measure.vi"("error in (no error)"=w382, "measurement type"=w308, "channel name"="1", "instrument handle"=w383) -> ("measurement"=w351:dbl)  [unwired: 5 in, 2 out]
        "VDD_cur, A" <- w351
        n206 = call <instrlib>:"niDCPower Measure.vi"("error in (no error)"=w355, "measurement type"=w308, "channel name"="0", "instrument handle"=w356) -> ("measurement"=w349:dbl)  [unwired: 5 in, 2 out]
        "VDPIX_cur, A" <- w349
        n207 = call <instrlib>:"niDCPower Measure.vi"("measurement type"=w308, "channel name"="1", "instrument handle"=w335) -> ("measurement"=w333:dbl)  [unwired: 6 in, 2 out]
        "VCC_cur, A" <- w333
        n208 = call <instrlib>:"niDCPower Measure.vi"("measurement type"=w308, "channel name"="0", "instrument handle"=w328) -> ("measurement"=w327:dbl)  [unwired: 6 in, 2 out]
        "DVDD_cur, A" <- w327
        n209 = call <instrlib>:"niDCPower Measure.vi"("measurement type"=w308, "channel name"="1", "instrument handle"=w313) -> ("measurement"=w314:dbl)  [unwired: 6 in, 2 out]
        "VDDA_cur, A" <- w314
        n210 = Wait (ms)(milliseconds to wait=u32 1) -> ()  [unwired: 1 out]
        n211 = Multiply(x=w333, y=1000.0) -> (x*y=→"VCC Chart":dbl)
        n212 = Multiply(x=w348, y=1000.0) -> (x*y=→"VDA Chart":dbl)
        n213 = Multiply(x=w351, y=1000.0) -> (x*y=→"VDD Chart":dbl)
        n214 = Multiply(x=w349, y=1000.0) -> (x*y=→"VDPIX Chart":dbl)
        n215 = Multiply(x=w327, y=1000.0) -> (x*y=→"DVDD Chart":dbl)
        n216 = Multiply(x=w314, y=1000.0) -> (x*y=→"VDDA Chart":dbl)
      }
      frame #1 {
      }
    }
  }
  n217 = while {
    tunnel: w1 -> [w392]
    tunnel: [w391] -> w31
    stop <- w402 stop-if-true
    n218 = call-poly <instrlib>:"niDMM Config Measurement.vi"("Range"=10.0, "Resolution"=0.001, "Function"=niDMM_Function."DC Volts", "instrument handle"=w392) -> ("error out"=w398:errorcluster, "instrument handle out"=w395:refnum<k15>)  [unwired: 6 in]
    n219 = call <instrlib>:"niDMM Read.vi"("error in (no error)"=w398, "instrument handle"=w395) -> ("Measurement"=w399:dbl, "instrument handle out"=w391:refnum<k15>)  [unwired: 7 in, 1 out]
    n220 = Multiply(x=w399, y=1000.0) -> (x*y=→"SEU, мВ":dbl)
    n221 = local read "Стоп"() -> (w402:bool)
    n222 = Wait (ms)(milliseconds to wait=u32 100) -> ()  [unwired: 1 out]
  }
  n223 = call <instrlib>:"niDMM Close.vi"("instrument handle"=w31) -> ()  [unwired: 10 in, 1 out]
  n224 = call <instrlib>:"niFgen Abort Generation.vi"("error in (no error)"=w12, "Instrument Handle"=w16) -> ("error out"=w29:errorcluster, "Instrument Handle Out"=w30:refnum<k15>)  [unwired: 8 in]
  n225 = call <instrlib>:"niFgen Close.vi"("error in (no error)"=w29, "Instrument Handle"=w30) -> ("error out"=w28:errorcluster)  [unwired: 9 in]
  n226 = call <vilib>:"Simple Error Handler.vi"("error in (no error)"=w28) -> ()  [unwired: 4 in, 5 out]
  n227 = Close File(refnum=w38) -> ()  [unwired: 1 in, 2 out]
  n228 = call <instrlib>:"niDCPower Close.vi"("instrument handle"=w35) -> ()  [unwired: 10 in, 1 out]
  n229 = call <instrlib>:"niDCPower Close.vi"("instrument handle"=w34) -> ()  [unwired: 10 in, 1 out]
  n230 = call <instrlib>:"niDCPower Close.vi"("instrument handle"=w33) -> ()  [unwired: 10 in, 1 out]
